vi "DM_Control_STED.vi"() -> ()   [LabVIEW 2014]
uses:
  DMControl_STED.ctl
  <vilib>/Utility/file.llb/Write To Spreadsheet File (DBL).vi
panel:
  in  "Exit":bool
  out "Voltage Map":dbl[][](graph)
  in  "Control":T1={"Type"=enum."Mirror", "Modes"=[{"Mode"="1", "Amplititude"=0.0}, {"Mode"="2", "Amplititude"=0.0}, {"Mode"="3", "Amplititude"=-0.999997086434591}, {"Mode"="4", "Amplititude"=1.5000119526293343}, {"Mode"="5", "Amplititude"=1.0000058955291342}, {"Mode"="6", "Amplititude"=1.654200285880384e-05}, {"Mode"="7", "Amplititude"=0.5000034787280048}, {"Mode"="8", "Amplititude"=5.348985710245131e-06}, {"Mode"="9", "Amplititude"=1.500005239264598}, {"Mode"="10", "Amplititude"=-0.49998827275038527}, {"Mode"="11", "Amplititude"=0.5000100463848842}, {"Mode"="12", "Amplititude"=6.713798753673702e-06}, {"Mode"="13", "Amplititude"=0.5000067992221375}, {"Mode"="14", "Amplititude"=-0.4999888820777417}, {"Mode"="15", "Amplititude"=-0.499999514659055}, {"Mode"="16", "Amplititude"=0.5000051964386535}, {"Mode"="17", "Amplititude"=-0.4999981572176452}, {"Mode"="18", "Amplititude"=0.5000009883738648}, {"Mode"="19", "Amplititude"=-0.4999927736672987}, {"Mode"="20", "Amplititude"=-0.4999895996219542}, {"Mode"="21", "Amplititude"=-0.999999228393673}, {"Mode"="22", "Amplititude"=0.5000038601801795}, {"Mode"="23", "Amplititude"=-0.4999907361054472}, {"Mode"="24", "Amplititude"=0.5000107727699616}, {"Mode"="25", "Amplititude"=0.5000003831379185}, {"Mode"="26", "Amplititude"=-1.4999933650813315}, {"Mode"="27", "Amplititude"=1.0602703816783579e-05}, {"Mode"="28", "Amplititude"=2.500005381391621}, {"Mode"="29", "Amplititude"=0.5000011193752751}, {"Mode"="30", "Amplititude"=9.489499053535159e-06}, {"Mode"="31", "Amplititude"=0.0}, {"Mode"="32", "Amplititude"=0.0}, {"Mode"="33", "Amplititude"=0.0}, {"Mode"="34", "Amplititude"=0.0}, {"Mode"="35", "Amplititude"=0.0}, {"Mode"="36", "Amplititude"=0.0}, {"Mode"="37", "Amplititude"=0.0}, {"Mode"="38", "Amplititude"=0.0}, {"Mode"="39", "Amplititude"=0.0}, {"Mode"="40", "Amplititude"=0.0}, {"Mode"="41", "Amplititude"=0.0}, {"Mode"="42", "Amplititude"=0.0}, {"Mode"="43", "Amplititude"=0.0}, {"Mode"="44", "Amplititude"=0.0}, {"Mode"="45", "Amplititude"=0.0}, {"Mode"="46", "Amplititude"=0.0}, {"Mode"="47", "Amplititude"=0.0}, {"Mode"="48", "Amplititude"=0.0}, {"Mode"="49", "Amplititude"=0.0}, {"Mode"="50", "Amplititude"=0.0}, {"Mode"="51", "Amplititude"=0.0}, {"Mode"="52", "Amplititude"=0.0}, {"Mode"="53", "Amplititude"=0.0}, {"Mode"="54", "Amplititude"=0.0}, {"Mode"="55", "Amplititude"=0.0}, {"Mode"="56", "Amplititude"=0.0}, {"Mode"="57", "Amplititude"=0.0}, {"Mode"="58", "Amplititude"=0.0}, {"Mode"="59", "Amplititude"=0.0}, {"Mode"="60", "Amplititude"=0.0}, {"Mode"="61", "Amplititude"=0.0}, {"Mode"="62", "Amplititude"=0.0}, {"Mode"="63", "Amplititude"=0.0}, {"Mode"="64", "Amplititude"=0.0}, {"Mode"="65", "Amplititude"=0.0}, {"Mode"="66", "Amplititude"=0.0}, {"Mode"="67", "Amplititude"=0.0}, {"Mode"="68", "Amplititude"=0.0}, {"Mode"="69", "Amplititude"=0.0}, {"Mode"="70", "Amplititude"=0.0}, {"Mode"="71", "Amplititude"=0.0}, {"Mode"="72", "Amplititude"=0.0}, {"Mode"="73", "Amplititude"=0.0}, {"Mode"="74", "Amplititude"=0.0}, {"Mode"="75", "Amplititude"=0.0}, {"Mode"="76", "Amplititude"=0.0}, {"Mode"="77", "Amplititude"=0.0}, {"Mode"="78", "Amplititude"=0.0}, {"Mode"="79", "Amplititude"=0.0}, {"Mode"="80", "Amplititude"=0.0}, {"Mode"="81", "Amplititude"=0.0}, {"Mode"="82", "Amplititude"=0.0}, {"Mode"="83", "Amplititude"=0.0}, {"Mode"="84", "Amplititude"=0.0}, {"Mode"="85", "Amplititude"=0.0}, {"Mode"="86", "Amplititude"=0.0}, {"Mode"="87", "Amplititude"=0.0}, {"Mode"="88", "Amplititude"=0.0}, {"Mode"="89", "Amplititude"=0.0}, {"Mode"="90", "Amplititude"=0.0}, {"Mode"="91", "Amplititude"=0.0}, {"Mode"="92", "Amplititude"=0.0}, {"Mode"="93", "Amplititude"=0.0}, {"Mode"="94", "Amplititude"=0.0}, {"Mode"="95", "Amplititude"=0.0}, {"Mode"="96", "Amplititude"=0.0}, {"Mode"="97", "Amplititude"=0.0}, {"Mode"="98", "Amplititude"=0.0}, {"Mode"="99", "Amplititude"=0.0}, {"Mode"="100", "Amplititude"=0.0}, {"Mode"="101", "Amplititude"=0.0}, {"Mode"="102", "Amplititude"=0.0}, {"Mode"="103", "Amplititude"=0.0}, {"Mode"="104", "Amplititude"=0.0}, {"Mode"="105", "Amplititude"=0.0}, {"Mode"="106", "Amplititude"=0.0}, {"Mode"="107", "Amplititude"=0.0}, {"Mode"="108", "Amplititude"=0.0}, {"Mode"="109", "Amplititude"=0.0}, {"Mode"="110", "Amplititude"=0.0}, {"Mode"="111", "Amplititude"=0.0}, {"Mode"="112", "Amplititude"=0.0}, {"Mode"="113", "Amplititude"=0.0}, {"Mode"="114", "Amplititude"=0.0}, {"Mode"="115", "Amplititude"=0.0}, {"Mode"="116", "Amplititude"=0.0}, {"Mode"="117", "Amplititude"=0.0}, {"Mode"="118", "Amplititude"=0.0}, {"Mode"="119", "Amplititude"=0.0}, {"Mode"="120", "Amplititude"=0.0}, {"Mode"="121", "Amplititude"=0.0}, {"Mode"="122", "Amplititude"=0.0}, {"Mode"="123", "Amplititude"=0.0}, {"Mode"="124", "Amplititude"=0.0}, {"Mode"="125", "Amplititude"=0.0}, {"Mode"="126", "Amplititude"=0.0}, {"Mode"="127", "Amplititude"=0.0}, {"Mode"="128", "Amplititude"=0.0}, {"Mode"="129", "Amplititude"=0.0}, {"Mode"="130", "Amplititude"=0.0}, {"Mode"="131", "Amplititude"=0.0}, {"Mode"="132", "Amplititude"=0.0}, {"Mode"="133", "Amplititude"=0.0}, {"Mode"="134", "Amplititude"=0.0}, {"Mode"="135", "Amplititude"=0.0}, {"Mode"="136", "Amplititude"=0.0}, {"Mode"="137", "Amplititude"=0.0}, {"Mode"="138", "Amplititude"=0.0}, {"Mode"="139", "Amplititude"=0.0}, {"Mode"="140", "Amplititude"=0.0}], "Apply Flat"=FALSE, "Save Map"=FALSE, "Clear Voltage"=FALSE, "Abberation Files"=0, "Scan "=FALSE} {"Abberation Files" items=["Ideal Modes"]; "Modes"."Amplititude" step=0.05}
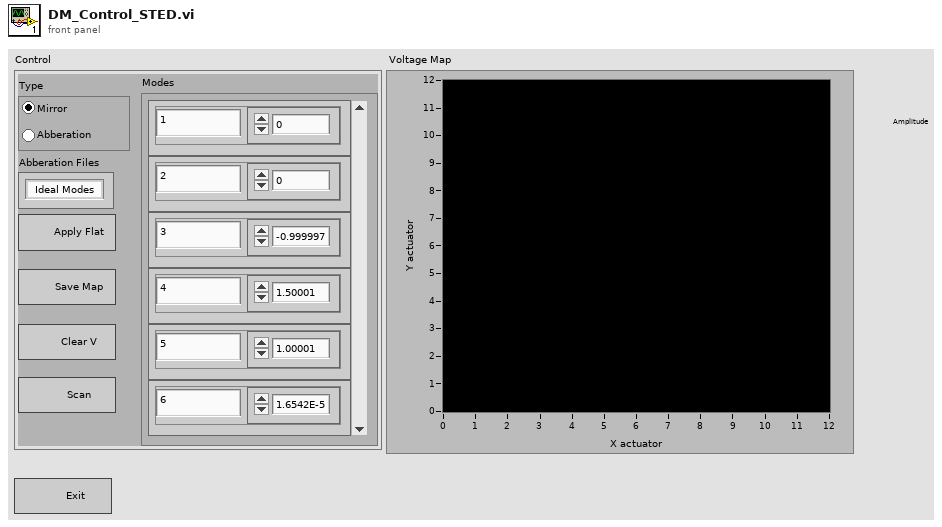
[diagram p1: front panel]
types:
  T1 = typedef "DMControl_STED.ctl" = cluster{"Type":enum32{"Mirror", "Abberation"}, "Modes":cluster{"Mode":string, "Amplititude":dbl}[], "Apply Flat":bool, "Save Map":bool, "Clear Voltage":bool, "Abberation Files":u16, "Scan ":bool}
  T2 = typedef "AbberationControl.ctl" = cluster{"Abberations":dbl[][], "Modes":i32[], "Abberations ID":string[], "Abberation Files":path[]}
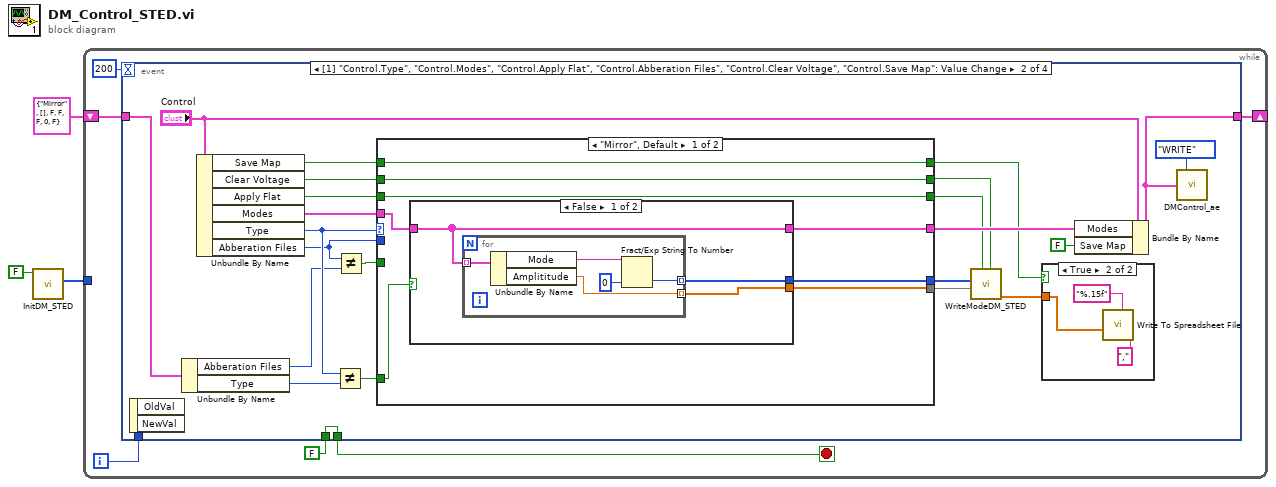
[diagram p0: block diagram]
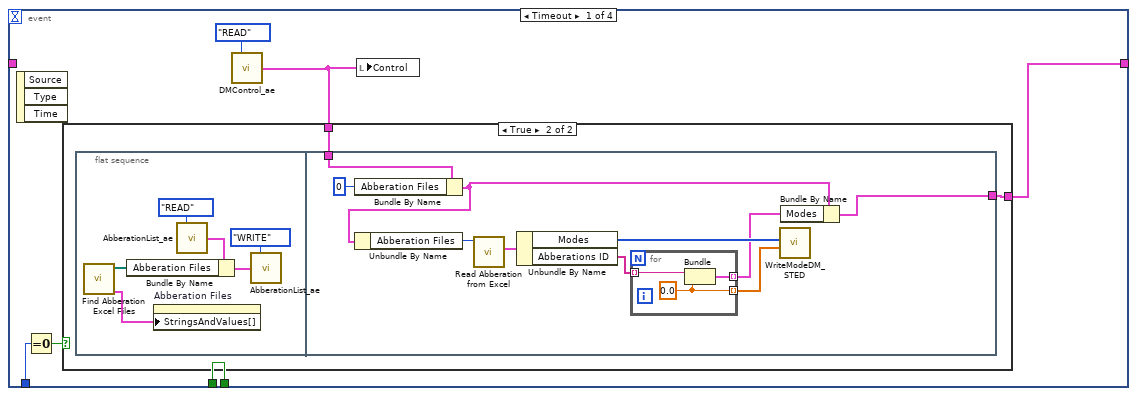
[diagram p2: hidden frame]
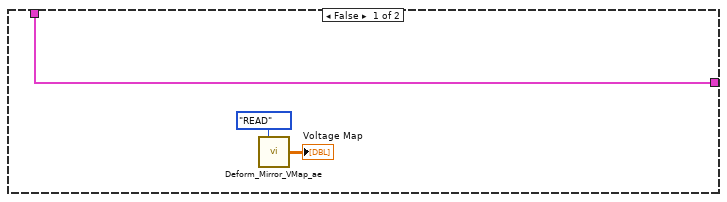
[diagram p3: hidden frame]
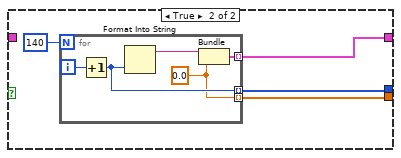
[diagram p5: hidden frame]
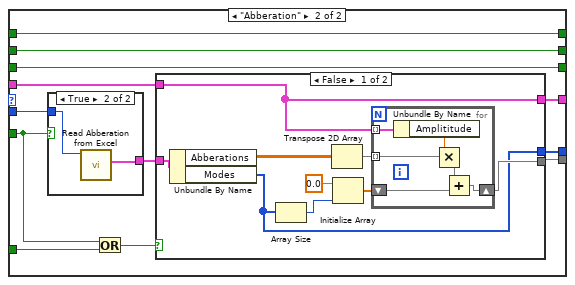
[diagram p6: hidden frame]
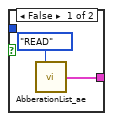
[diagram p7: hidden frame]
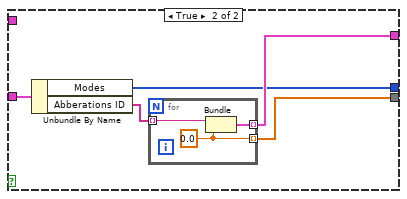
[diagram p8: hidden frame]
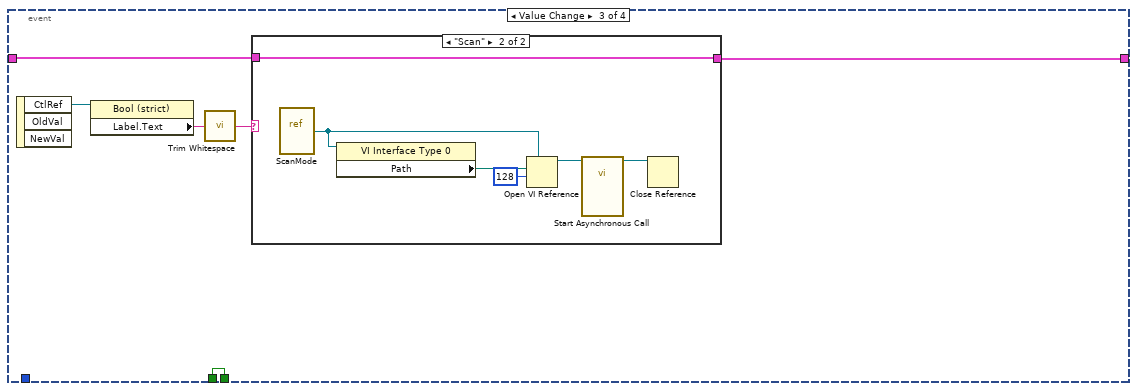
[diagram p9: hidden frame]
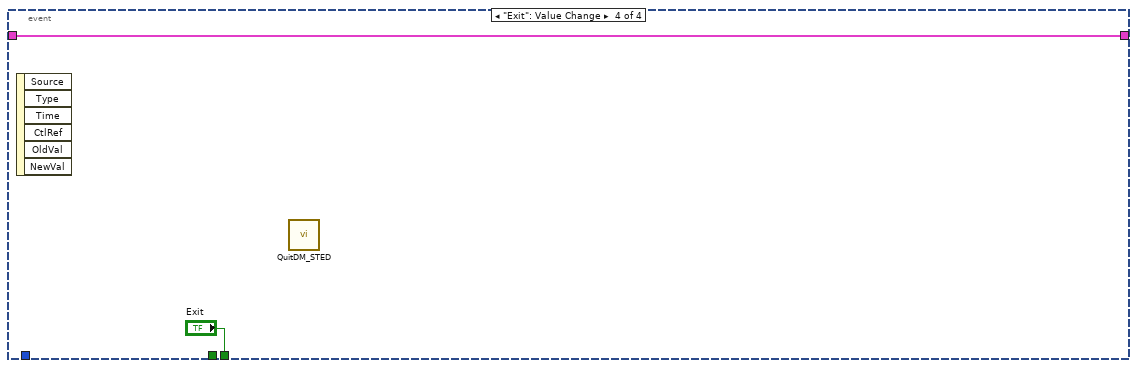
[diagram p11: hidden frame]
diagram:
  n1 = call "InitDM_STED.vi"("BM Flat"=FALSE) -> ("IDs"=w3:i32[])  [unwired: 9 in, 1 out]
  n2 = while {
    shift-right: [w6] -> _
    shift-left: T1 {"Type"=enum."Mirror", "Modes"=[], "Apply Flat"=FALSE, "Save Map"=FALSE, "Clear Voltage"=FALSE, "Abberation Files"=0, "Scan "=FALSE} ("Control") -> [w7]
    tunnel: w3 -> [_]
    i -> [w4]
    stop <- w9 stop-if-true
    n3 = event shown="[1] \"Control.Type\", \"Control.Modes\", \"Control.Apply Flat\", \"Control.Abberation Files\", \"Control.Clear Voltage\", \"Control.Save Map\": Value Change" {
      selector: _ -> [_ _ _ _]
      dyn-events: _ -> [_ _ _ _]
      timeout: 200 -> [_ _ _ _]
      tunnel: [w15 w62 w132 "Exit"] -> w9
      tunnel: FALSE -> [w15 w62 w132 _]
      tunnel: w7 -> [_ w52 w134 w143]
      tunnel: [w14 w44 w133 w143] -> w6
      tunnel: w4 -> [w13 _ _ _]
      event Timeout {
        n4 = event-data() -> ()  [unwired: 1 in, 3 out]
        n5 = Equal To 0?(x=w13) -> (x = 0?=w12:bool)
        n6 = call "DMControl_ae.vi"("Enum"=enum16{"WRITE", "READ"}."READ") -> ("Abberation Cluster Out"=w10:T1)  [unwired: 14 in]
        n7 = case shown="True" w12 {
          tunnel: w10 -> [w16 w20]
          tunnel: [w16 w19] -> w14
          frame False {
            n8 = call "Deform_Mirror_VMap_ae.vi"("Action"=enum16{"WRITE", "READ"}."READ") -> ("V Map Out"=→"Voltage Map":dbl[][])  [unwired: 14 in]
          }
          frame True {
            n9 = flat-sequence {
              tunnel: w20 -> [w31]
              tunnel: [w27] -> w19
              frame #0 {
                n10 = call "Find Abberation Excel Files.vi"() -> ("Ring Menu"=w21:cluster{"result string":string, i32}[], "Abberation File Paths"=w24:path[])  [unwired: 10 in]
                n11 = property on="Abberation Files" class="Ring (strict)"("StringsAndValues[]"=w21) -> ()  [unwired: 2 in, 2 out]
                n12 = call "AbberationList_ae.vi"("Enum"=enum16{"WRITE", "READ"}."READ") -> ("Abberation Cluster Out"=w25:T2)  [unwired: 14 in]
                n13 = Bundle By Name(cluster=w25, "Abberation Files"=w24) -> (w22:T2)
                n14 = call "AbberationList_ae.vi"("Enum"=enum16{"WRITE", "READ"}."WRITE", "Abberation Cluster In"=w22) -> ()  [unwired: 13 in, 1 out]
              }
              frame #1 {
                n15 = Bundle By Name(cluster=w31, "Abberation Files"=u16 0) -> (w29:T1)
                n16 = Unbundle By Name(w29) -> ("Abberation Files"=w32:u16)
                n17 = call "Read Abberation from Excel.vi"("Ring"=w32) -> ("output cluster"=w35:T2)  [unwired: 8 in]
                n18 = Unbundle By Name(w35) -> ("Modes"=w34:i32[], "Abberations ID"=w36:string[])
                n19 = for {
                  tunnel: w36 -> [w37] mode=indexing
                  tunnel: [w39] -> w33 mode=indexing
                  tunnel: [w38] -> w28 mode=indexing
                  w39 = 0.0
                  n20 = Bundle(w37, w39) -> (w38:cluster{string, dbl})  [unwired: 1 in]
                }
                n21 = call "WriteModeDM_STED.vi"("Amplitudes"=w33, "Modes"=w34) -> ()  [unwired: 8 in, 2 out]
                n22 = Bundle By Name(cluster=w29, "Modes"=w28) -> (w27:T1)
              }
            }
          }
        }
        n23 = local write "Control"(w10) -> ()
      }
      event Value Change {
        n24 = event-data() -> ()  [unwired: 1 in, 2 out]
        n25 = Unbundle By Name(w52) -> ("Abberation Files"=w48:u16, "Type"=w51:enum32{"Mirror", "Abberation"})
        n26 = Unbundle By Name("Control") -> ("Save Map"=w43:bool, "Clear Voltage"=w53:bool, "Apply Flat"=w55:bool, "Modes"=w61:cluster{"Mode":string, "Amplititude":dbl}[], "Type"=w49:enum32{"Mirror", "Abberation"}, "Abberation Files"=w46:u16)
        n27 = Not Equal?(x=w49, y=w51) -> (x != y?=w50:bool)
        n28 = Not Equal?(x=w46, y=w48) -> (x != y?=w47:bool)
        n29 = case shown="\"Mirror\", Default" w49 {
          tunnel: w61 -> [w67 w97]
          tunnel: [w73 w100] -> w60
          tunnel: [w72 w99] -> w59
          tunnel: [w71 w98] -> w58
          tunnel: w55 -> [w70 w102]
          tunnel: [w70 w102] -> w57
          tunnel: [w69 w101] -> w54
          tunnel: w53 -> [w69 w101]
          tunnel: w50 -> [w68 w95]
          tunnel: w47 -> [_ w94]
          tunnel: w46 -> [_ w92]
          tunnel: [w66 w91] -> w42
          tunnel: w43 -> [w66 w91]
          frame "Mirror", Default {
            n30 = case shown="False" w68 {
              tunnel: [w74 w82] -> w73
              tunnel: [w76 w85] -> w72
              tunnel: [w75 w84] -> w71
              tunnel: w67 -> [w74 _]
              frame False {
                n31 = for {
                  tunnel: w74 -> [w81] mode=indexing
                  tunnel: [w78] -> w76 mode=indexing
                  tunnel: [w77] -> w75 mode=indexing
                  n32 = Unbundle By Name(w81) -> ("Mode"=w79:string, "Amplititude"=w77:dbl)
                  n33 = Fract/Exp String To Number(string=w79, default (0 dbl)=0) -> (number=w78:i32)  [unwired: 2 in, 1 out]
                }
              }
              frame True {
                n34 = for {
                  N: 140 -> [_]
                  tunnel: [w90] -> w85 mode=indexing
                  tunnel: [w88] -> w84 mode=indexing
                  tunnel: [w87] -> w82 mode=indexing
                  i -> [w86]
                  w88 = 0.0 ("input 1")
                  n35 = Increment(x=w86) -> (x+1=w90:i32)
                  n36 = Format Into String(w90) -> (resulting string=w89:string)  [unwired: 3 in, 1 out]
                  n37 = Bundle(w89, "input 1"=w88) -> (w87:cluster{string, "input 1":dbl})  [unwired: 1 in]
                }
              }
            }
          }
          frame "Abberation" {
            n38 = case shown="True" w94 {
              tunnel: [w103 w105] -> w96
              tunnel: w92 -> [_ w106]
              frame False {
                n39 = call "AbberationList_ae.vi"("Enum"=enum16{"WRITE", "READ"}."READ") -> ("Abberation Cluster Out"=w103:T2)  [unwired: 14 in]
              }
              frame True {
                n40 = call "Read Abberation from Excel.vi"("Ring"=w106) -> ("output cluster"=w105:T2)  [unwired: 8 in]
              }
            }
            n41 = Or(x=w94, y=w95) -> (x .or. y?=w93:bool)
            n42 = case shown="False" w93 {
              tunnel: [w107 w126] -> w100
              tunnel: [w110 w125] -> w99
              tunnel: [w112 w124] -> w98
              tunnel: w97 -> [w107 _]
              tunnel: w96 -> [w115 w123]
              frame False {
                n43 = Unbundle By Name(w115) -> ("Abberations"=w114:dbl[][], "Modes"=w110:i32[])
                n44 = Array Size(array=w110) -> (size(s)=w109:i32)
                n45 = Transpose 2D Array(2D array=w114) -> (transposed array=w113:dbl[][])
                n46 = Initialize Array(0.0 ("element"), w109) -> (w108:dbl[])
                n47 = for {
                  tunnel: w107 -> [w120] mode=indexing
                  tunnel: w113 -> [w121] mode=indexing
                  shift-right: [w118] -> w112
                  shift-left: w108 -> [w116]
                  n48 = Unbundle By Name(w120) -> ("Amplititude"=w119:dbl)
                  n49 = Multiply(x=w119, y=w121) -> (x*y=w117:dbl[])
                  n50 = Add(x=w117, y=w116) -> (x+y=w118:dbl[])
                }
              }
              frame True {
                n51 = Unbundle By Name(w123) -> ("Modes"=w125:i32[], "Abberations ID"=w122:string[])
                n52 = for {
                  tunnel: w122 -> [w127] mode=indexing
                  tunnel: [w129] -> w124 mode=indexing
                  tunnel: [w128] -> w126 mode=indexing
                  w129 = 0.0
                  n53 = Bundle(w127, w129) -> (w128:cluster{string, dbl})  [unwired: 1 in]
                }
              }
            }
          }
        }
        n54 = call "WriteModeDM_STED.vi"("ClearV"=w54, "Flat On"=w57, "Amplitudes"=w58, "Modes"=w59) -> ("V Map"=w40:dbl[])  [unwired: 6 in, 1 out]
        n55 = case shown="True" w42 {
          tunnel: w40 -> [_ w64]
          frame False {
          }
          frame True {
            n56 = call-poly <vilib>:"Write To Spreadsheet File.vi"("delimiter (\\t)"="," ("delimiter (\\t)"), "format (%.3f)"="%.15f", "1D data"=w64) -> ()  [unwired: 5 in, 1 out]
          }
        }
        n57 = Bundle By Name(cluster="Control", "Modes"=w60, "Save Map"=FALSE) -> (w44:T1)
        n58 = call "DMControl_ae.vi"("Enum"=enum16{"WRITE", "READ"}."WRITE", "Control"=w44) -> ()  [unwired: 13 in, 1 out]
      }
      event Value Change {
        n59 = event-data() -> ("CtlRef"=w135:refnum<vi>)  [unwired: 1 in, 2 out]
        n60 = property class="Bool (strict)"(reference=w135) -> ("Label.Text"=w131:string)  [unwired: 1 in, 2 out]
        n61 = call <vilib>:"Trim Whitespace.vi"("string"=w131) -> ("trimmed string"=w130:string)  [unwired: 1 in]
        n62 = case shown="\"Scan\"" w130 {
          tunnel: w134 -> [w136 w142]
          tunnel: [w136 w142] -> w133
          frame Default {
          }
          frame "Scan" {
            n63 = vi-ref "ScanMode.vi"() -> (w138:refnum<vi>)
            n64 = property class="VI Interface Type 0"(reference=w138) -> ("Path"=w140:path)  [unwired: 1 in, 2 out]
            n65 = Open VI Reference(type specifier VI Refnum (for type only)=w138, vi path=w140, options=128) -> (vi reference=w139:refnum<vi>)  [unwired: 3 in, 1 out]
            n66 = call-by-ref "Start Asynchronous Call"(reference=w139) -> (reference out=w137:refnum<vi>)  [unwired: 13 in, 1 out]
            n67 = Close Reference(reference=w137) -> ()  [unwired: 1 in, 1 out]
          }
        }
      }
      event "Exit": Value Change {
        n68 = event-data() -> ()  [unwired: 1 in, 6 out]
        n69 = call "QuitDM_STED.vi"() -> ()  [unwired: 12 in]
      }
    }
  }
